vi "get Julia ZMQ server path.vi"(8 "error in (no error)":errorcluster, 11 "Julia ZMQ server file name":string="ZMQ-testserver2.jl") -> (0 "error out":errorcluster, 2 "package base path":path, 3 "Julia ZMQ server file path":path)   [LabVIEW 2018, in "LV-Julia_ZMQ-Roundtrip_lib.lvlib"]
uses:
  LV-Julia_ZMQ-Roundtrip_lib.lvlib
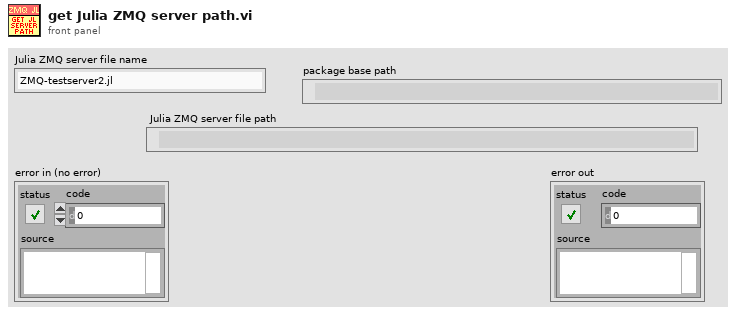
[diagram p1: front panel]
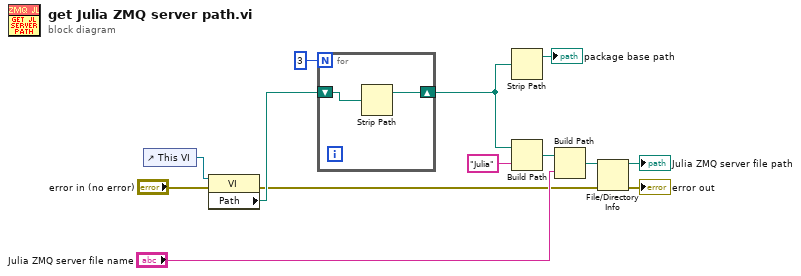
[diagram p0: block diagram]
diagram:
  n1 = control-ref of="This VI"() -> (w13:refnum<vi>)
  n2 = property class="VI"(reference=w13, error in="error in (no error)") -> (error out=w6:errorcluster, "Path"=w11:path)  [unwired: 1 out]
  n3 = for {
    N: 3 -> [_]
    shift-right: [w14] -> w1
    shift-left: w11 -> [w15]
    n4 = Strip Path(path=w15) -> (stripped path=w14:path)  [unwired: 1 out]
  }
  n5 = Strip Path(path=w1) -> (stripped path=→"package base path":path)  [unwired: 1 out]
  n6 = Build Path(base path=w1, name or relative path="Julia") -> (appended path=w10:path)
  n7 = Build Path(base path=w10, name or relative path="Julia ZMQ server file name") -> (appended path=w7:path)
  n8 = File/Directory Info(path=w7, error in=w6) -> (path out=→"Julia ZMQ server file path":path, error out=→"error out":errorcluster)  [unwired: 5 out]
